vi "Actor Core.vi"(8 "error in":errorcluster, 11 "Client in":refnum<class "Client.lvclass">) -> (0 "error out":errorcluster, 3 "Actor out":refnum<class "Actor.lvclass">)   [LabVIEW 2016, in "Client.lvlib" / "Client.lvclass"]
doc: "(<B>Filename</B>: Actor Framework.lvlib:Actor.lvclass:Actor Core.vi)\n\nReceives messages to the actor, reacts to them, and initiates any error handling that may shut the actor down.\n\nDescendant classes may override this VI to append parallel tasks for the actor to complete while it handles messages. Overrides use the Call Parent Method node."
uses:
  Client.lvclass
  <vilib>/ActorFramework/Actor/Actor.lvclass
  <vilib>/NI/STM/SubVIs/MetaDataElement.ctl
  <vilib>/NI/STM/UDP/UDP Write Options.ctl
  <vilib>/NI/STM/UDP/UDP Read Options.ctl
  Client.lvclass/Client.ctl
  <vilib>/NI/STM/TCP/Write Meta Data (TCP Ref).vi
  <vilib>/NI/STM/TCP/Get Connection Reference (TCP).vi
  <vilib>/NI/STM/UDP/Write Meta Data (UDP Ref).vi
  <vilib>/NI/STM/UDP/Get Connection Reference (UDP).vi
  <vilib>/NI/STM/UDP/Write Meta Data (UDP Clst).vi
  <vilib>/NI/STM/UDP/Write Message (UDP).vi
  <vilib>/NI/STM/UDP/Read Message (UDP).vi
  <vilib>/NI/STM/TCP/Write Meta Data (TCP Clst).vi
  <vilib>/NI/STM/TCP/Write Message (TCP).vi
  <vilib>/NI/STM/NI STM.lvlib
panel:
  in  "port":u16=55555
  out "Array":dbl[](array[numeric])
  out "ID string":string
  in  "stop":bool
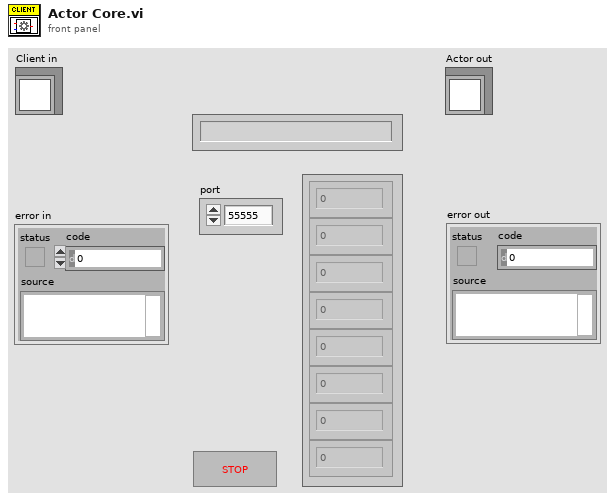
[diagram p1: front panel]
types:
  T1 = typedef "NI STM.lvlib/MetaDataElement.ctl" = string
  T2 = typedef "NI STM.lvlib/TCP Connection Info.ctl" = cluster{"connection ID":refnum<k5>, "meta data":T1[]}
  T3 = typedef "NI STM.lvlib/UDP Connection Info.ctl" = cluster{"connection ID":refnum<k16>, "meta data":T1[]}
  T4 = typedef "NI STM.lvlib/UDP Read Options.ctl" = cluster{"ignore timeout error":bool, "timeout ms (1000)":i32, "max size (548)":i32}
  T5 = typedef "NI STM.lvlib/UDP Write Options.ctl" = cluster{"ignore timeout error":bool, "timeout ms (1000)":i32}
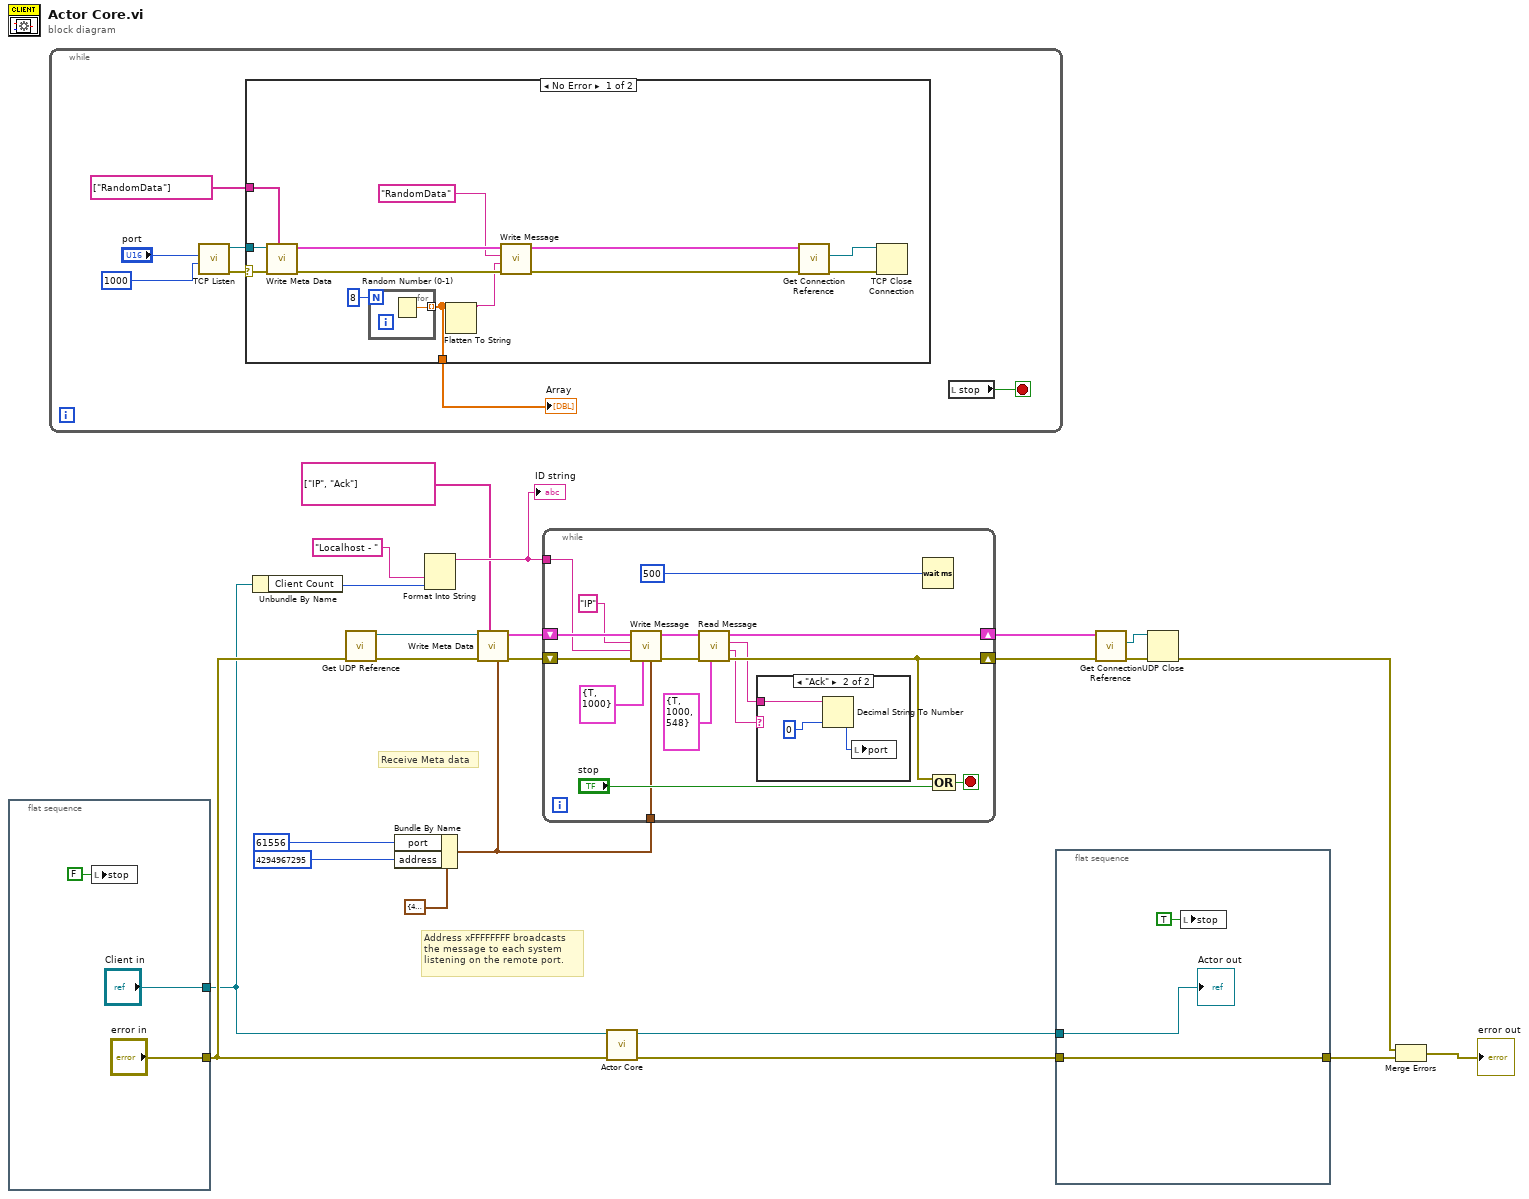
[diagram p0: block diagram]
diagram:
  # "Address xFFFFFFFF broadcasts\nthe message to each system\nlistening on the remote port."
  # "Receive Meta data"
  n1 = flat-sequence {
    tunnel: ["error in"] -> w11
    tunnel: ["Client in"] -> w10
    frame #0 {
      n2 = local write "stop"(FALSE ("stop")) -> ()
    }
  }
  n3 = while {
    stop <- w28 stop-if-true
    n4 = call <vilib>:"TCP Listen.vi"("timeout ms (wait forever: -1)"=1000, "port"="port") -> ("error out"=w31:errorcluster, "connection ID"=w32:refnum<k5>)  [unwired: 2 in, 6 out]
    n5 = case shown="No Error" w31 {
      selector: w31 -> [w45 _]
      tunnel: w32 -> [w46 _]
      tunnel: T1[] ["RandomData"] ("Meta data") -> [w38 _]
      tunnel: [w34 _] -> w27
      frame No Error {
        n6 = call-poly <vilib>:"Write Meta Data.vi"("meta data"=w38, "error in"=w45, "connection ID"=w46) -> ("error out"=w43:errorcluster, "connection info out"=w44:T2)  [unwired: 2 in, 5 out]
        n7 = for {
          N: 8 -> [_]
          tunnel: [w47] -> w34 mode=indexing
          n8 = Random Number (0-1)() -> (number: 0 to 1=w47:dbl)
        }
        n9 = Flatten To String(anything=w34) -> (data string=w35:string)  [unwired: 1 in, 4 out]
        n10 = call-poly <vilib>:"Write Message.vi"("error in"=w43, "data"=w35, "name"="RandomData" ("Name"), "connection info in"=w44) -> ("error out"=w40:errorcluster, "connection info out"=w42:T2)  [unwired: 1 in, 5 out]
        n11 = call-poly <vilib>:"Get Connection Reference.vi"("error in"=w40, "connection info in"=w42) -> ("error out"=w39:errorcluster, "connection ID out"=w41:refnum<k5>)  [unwired: 8 out]
        n12 = TCP Close Connection(connection ID=w41, error in (no error)=w39) -> ()  [unwired: 3 out]
      }
      frame Error {
      }
    }
    "Array" <- w27
    n13 = local read "stop"() -> (w28:bool)
  }
  n14 = Unbundle By Name(w10) -> ("Client Count"=w9:i32)
  n15 = call "Get UDP Reference.vi"("error in (no error)"=w11) -> ("error out"=w14:errorcluster, "UDP Network Connection"=w13:refnum<k16>)  [unwired: 9 in]
  n16 = Bundle By Name(cluster=cluster{"address":u32, "port":u16} {"address"=4294967295, "port"=0} ("Address"), "port"=u16 61556 ("remote port"), "address"=u32 4294967295) -> (w2:cluster{"address":u32, "port":u16})
  n17 = Format Into String("Localhost - ", w9) -> (resulting string=w7:string)  [unwired: 3 in, 1 out]
  "ID string" <- w7
  n18 = call-poly <vilib>:"Write Meta Data.vi"("address"=w2, "meta data"=T1[] ["IP", "Ack"], "error in"=w14, "connection ID"=w13) -> ("error out"=w16:errorcluster, "connection info out"=w15:T3)  [unwired: 6 in]
  n19 = while {
    shift-right: [w51] -> w17
    shift-left: w15 -> [w63]
    shift-right: [w53] -> w1
    shift-left: w16 -> [w62]
    tunnel: w2 -> [w59]
    tunnel: w7 -> [w56]
    stop <- w61 stop-if-true
    n20 = call-poly <vilib>:"Write Message.vi"("address"=w59, "options"=T5 {"ignore timeout error"=TRUE, "timeout ms (1000)"=1000}, "error in"=w62, "data"=w56, "name"="IP" ("Name"), "connection info in"=w63) -> ("error out"=w58:errorcluster, "connection info out"=w52:T3)  [unwired: 1 in, 3 out]
    n21 = call-poly <vilib>:"Read Message.vi"("options"=T4 {"ignore timeout error"=TRUE, "timeout ms (1000)"=1000, "max size (548)"=548}, "error in"=w58, "connection info in"=w52) -> ("error out"=w53:errorcluster, "name"=w49:T1, "data string"=w48:string, "connection info out"=w51:T3)  [unwired: 3 in, 2 out]
    n22 = case shown="\"Ack\"" w49 {
      tunnel: w48 -> [_ w66]
      frame Default {
      }
      frame "Ack" {
        n23 = Decimal String To Number(string=w66, default (0L)=u16 0 ("port")) -> (number=w64:u16)  [unwired: 1 in, 1 out]
        n24 = local write "port"(w64) -> ()
      }
    }
    n25 = Wait (ms)(milliseconds to wait=u32 500) -> ()  [unwired: 1 out]
    n26 = Compound Arithmetic op=OR(w53, "stop") -> (w61:bool)
  }
  n27 = call-parent "Actor Core.vi"("error in"=w11, "Actor in"=w10) -> ("error out"=w23:errorcluster, "Actor out"=w22:refnum<class "Actor.lvclass">)  [unwired: 8 in]
  n28 = flat-sequence {
    tunnel: w23 -> [w67]
    tunnel: w22 -> [w69]
    tunnel: [w67] -> w6
    frame #0 {
      n29 = local write "stop"(TRUE ("stop")) -> ()
      "Actor out" <- w69
    }
  }
  n30 = call-poly <vilib>:"Get Connection Reference.vi"("error in"=w1, "connection info in"=w17) -> ("error out"=w19:errorcluster, "connection ID"=w18:refnum<k16>)  [unwired: 8 out]
  n31 = UDP Close(connection ID=w18, 8:w19) -> (error out=w4:errorcluster)  [unwired: 1 out]
  n32 = Merge Errors(w4, w6) -> (→"error out":errorcluster)
